vi "Rectangle Comparison.vi"(6 "Line Border":cluster{"Top":dbl, "Bottom":dbl}={"Top"=6.0, "Bottom"=1.0}, 9 "Second":dbl[](array[numeric]), 11 "First":dbl[](array[numeric])) -> (0 "Rect":T1, 1 "Line":T1, 3 "Scores":T2)   [LabVIEW 2016]
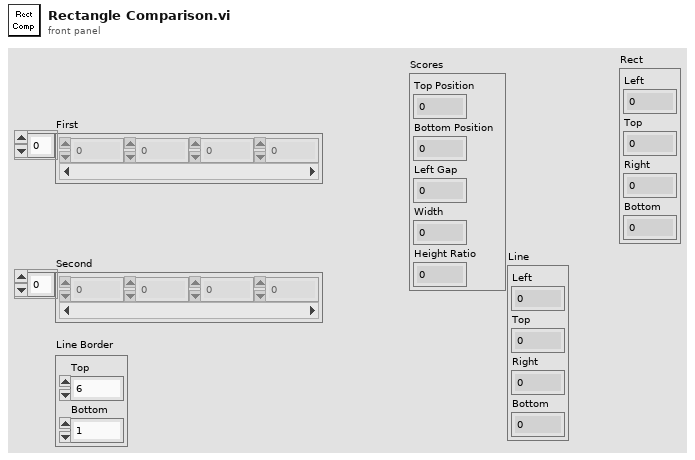
[diagram p1: front panel]
types:
  T1 = cluster{"Left":dbl, "Top":dbl, "Right":dbl, "Bottom":dbl}
  T2 = cluster{"Top Position":dbl, "Bottom Position":dbl, "Left Gap":dbl, "Width":dbl, "Height Ratio":dbl}
  T3 = cluster{"[0]":dbl, "[1]":dbl, "[2]":dbl, "[3]":dbl}
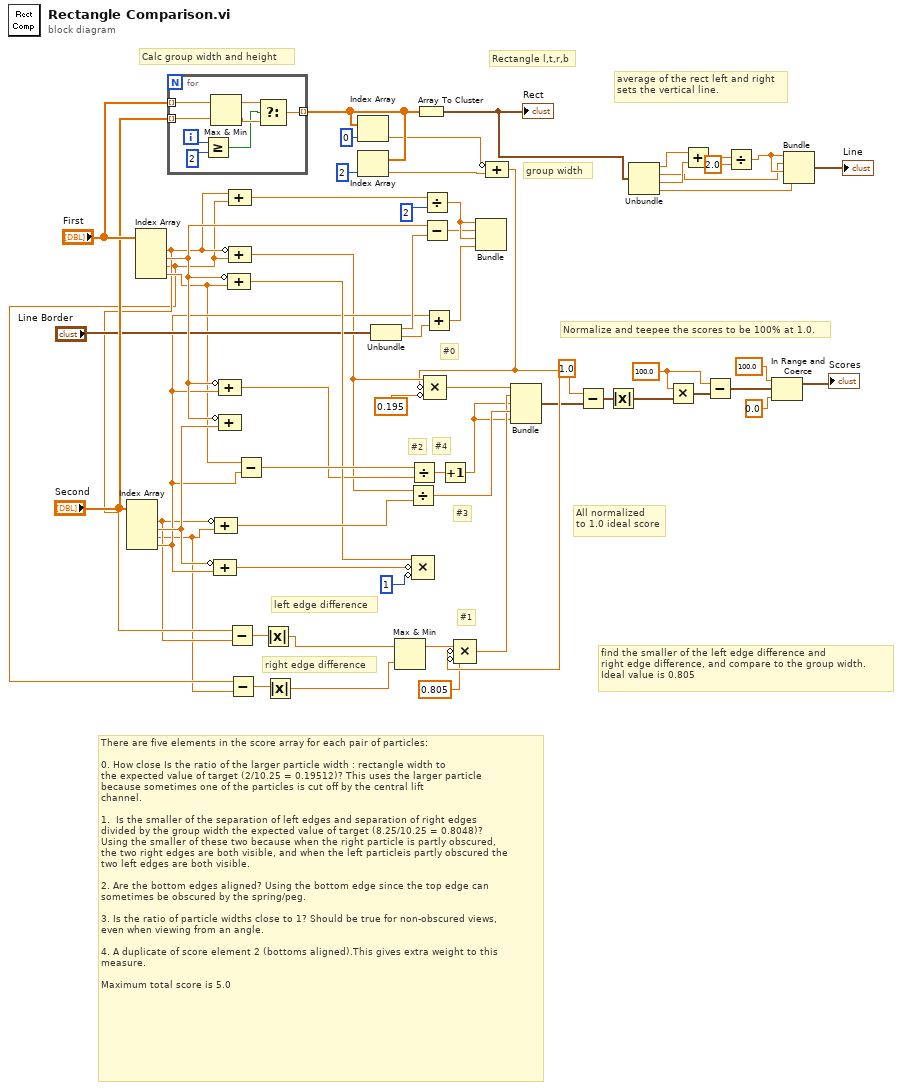
[diagram p0: block diagram]
diagram:
  w46 = 100.0 ("x/y")
  # "#4"
  # "#3"
  # "#2"
  # "#1"
  # "#0"
  # "There are five elements in the score array for each pair of particles:\n\n0. How close Is the ratio of the larger particle width : rectangle width to \nthe expected value of target (2/10.25 = 0.19512)? This uses the larger particle \nbecause sometimes one of the particles is cut off by the central lift \nchannel.\n\n1.  Is the smaller of the separation of left edges and separation of right edges\ndivided by the group width the expected value of target (8.25/10.25 = 0.8048)?\nUsing the smaller of these two because when the right particle is partly obscured,\nthe two right edges are both visible, and when the left particleis partly obscured the \ntwo left edges are both visible.\n\n2. Are the bottom edges aligned? Using the bottom edge since the top edge can \nsometimes be obscured by the spring/peg.\n\n3. Is the ratio of particle widths close to 1? Should be true for non-obscured views,\neven when viewing from an angle.\n\n4. A duplicate of score element 2 (bottoms aligned).This gives extra weight to this\nmeasure.\n\nMaximum total score is 5.0"
  # "average of the rect left and right\nsets the vertical line."
  # "find the smaller of the left edge difference and \nright edge difference, and compare to the group width.\nIdeal value is 0.805"
  # "group width"
  # "right edge difference"
  # "left edge difference"
  # "All normalized\nto 1.0 ideal score"
  # "Normalize and teepee the scores to be 100% at 1.0."
  # "Calc group width and height"
  # "Rectangle l,t,r,b"
  n1 = Index Array(array="Second") -> (element #1=w23:dbl, element #2=w39:dbl, element #3=w19:dbl, element #4=w33:dbl)  [unwired: 4 in]
  n2 = Index Array(array="First") -> (element #1=w24:dbl, element #2=w38:dbl, element #3=w20:dbl, element #4=w32:dbl)  [unwired: 4 in]
  n3 = for {
    tunnel: "First" -> [w70] mode=indexing
    tunnel: "Second" -> [w69] mode=indexing
    tunnel: [w63] -> w28 mode=indexing
    i -> [w67]
    n4 = Greater Or Equal?(x=w67, y=2) -> (x >= y?=w64:bool)
    n5 = Max & Min(x=w70, y=w69) -> (max(x,y)=w66:dbl, min(x,y)=w65:dbl)
    n6 = Select(t=w66, s=w64, f=w65) -> (s? t:f=w63:dbl)
  }
  n7 = Compound Arithmetic op=ADD(invert w39, w33) -> (w61:dbl)
  n8 = Compound Arithmetic op=ADD(invert w23, w19) -> (w62:dbl)
  n9 = Compound Arithmetic op=ADD(invert w38, w33) -> (w31:dbl)
  n10 = Compound Arithmetic op=ADD(invert w38, w39) -> ()  [unwired: 1 out]
  n11 = Subtract(x=w24, y=w23) -> (x-y=w22:dbl)
  n12 = Compound Arithmetic op=ADD(invert w38, w32) -> (w40:dbl)
  n13 = Subtract(x=w20, y=w19) -> (x-y=w21:dbl)
  n14 = Compound Arithmetic op=ADD(w24, w20) -> (w56:dbl)
  n15 = Compound Arithmetic op=ADD(invert w24, w20) -> (w30:dbl)
  n16 = Subtract(x=w32, y=w33) -> (x-y=w60:dbl)
  n17 = Absolute Value(x=w22) -> (abs(x)=w18:dbl)
  n18 = Absolute Value(x=w21) -> (abs(x)=w17:dbl)
  n19 = Index Array(array=w28, index=0) -> (element=w26:dbl)
  n20 = Index Array(array=w28, index=2) -> (element=w27:dbl)
  n21 = Unbundle("Line Border") -> ("Top"=w34:dbl, "Bottom"=w35:dbl)
  n22 = Max & Min(x=w18, y=w17) -> (max(x,y)=w16:dbl)  [unwired: 1 out]
  n23 = Divide(x=w30, y=w62) -> (x/y=w58:dbl)
  n24 = Divide(x=w60, y=w31) -> (x/y=w57:dbl)
  n25 = Compound Arithmetic op=MULTIPLY(w40, invert w61, invert 1) -> ()  [unwired: 1 out]
  n26 = Array To Cluster(array=w28) -> (cluster=w9:T3)
  "Rect" <- w9
  n27 = Divide(x=w56, y=2) -> (x/y=w55:dbl)
  n28 = Subtract(x=w38, y=w34) -> (x-y=w54:dbl)
  n29 = Add(x=w33, y=w35) -> (x+y=w50:dbl)
  n30 = Increment(x=w57) -> (x+1=w10:dbl)
  n31 = Bundle(w55, w54, w55, w50) -> ()  [unwired: 1 in, 1 out]
  n32 = Compound Arithmetic op=ADD(invert w26, w27) -> (w15:dbl)
  n33 = Compound Arithmetic op=MULTIPLY(w30, invert w15, invert 0.195 ("y")) -> (w59:dbl)
  n34 = Compound Arithmetic op=MULTIPLY(w16, invert w15, invert 0.805 ("y")) -> (w13:dbl)
  n35 = Bundle(w59, w13, w10, w58, w10) -> (w12:cluster{dbl, dbl, dbl, dbl, dbl})  [unwired: 1 in]
  n36 = Subtract(x=1.0 ("y"), y=w12) -> (x-y=w44:cluster{dbl, dbl, dbl, dbl, dbl})
  n37 = Absolute Value(x=w44) -> (abs(x)=w47:cluster{dbl, dbl, dbl, dbl, dbl})
  n38 = Unbundle(w9) -> ("[0]"=w8:dbl, "[1]"=w2:dbl, "[2]"=w7:dbl, "[3]"=w1:dbl)
  n39 = Multiply(x=w46, y=w47) -> (x*y=w48:cluster{dbl, dbl, dbl, dbl, dbl})
  n40 = Add(x=w8, y=w7) -> (x+y=w6:dbl)
  n41 = Subtract(x=w46, y=w48) -> (x-y=w43:cluster{dbl, dbl, dbl, dbl, dbl})
  n42 = Divide(x=w6, y=2.0) -> (x/y=w3:dbl)
  n43 = In Range and Coerce(upper limit=100.0, x=w43, lower limit=0.0) -> (coerced(x)=→"Scores":cluster{dbl, dbl, dbl, dbl, dbl})  [unwired: 1 out]
  n44 = Bundle(w3, "[1]"=w2, w3, "[3]"=w1) -> (→"Line":cluster{dbl, "[1]":dbl, dbl, "[3]":dbl})  [unwired: 1 in]
